vi "SortControlsColumn__slk_mt.vi"(8 "error in (no error)":errorcluster, 9 "Index":i32, 10 "Area Scale":T1, 11 "Controls":refnum<vi>[](array[refnum])) -> (0 "error out":errorcluster, 1 "Index":u32[](array[numeric]))   [LabVIEW 2015, in "Lazyboots Menu Tool.lvlib"]
uses:
  <vilib>/Utility/miscctls.llb/LVRectTypeDef.ctl
  <vilib>/SLK/Lazyboots Menu Tool/Library/Lazyboots Menu Tool.lvlib
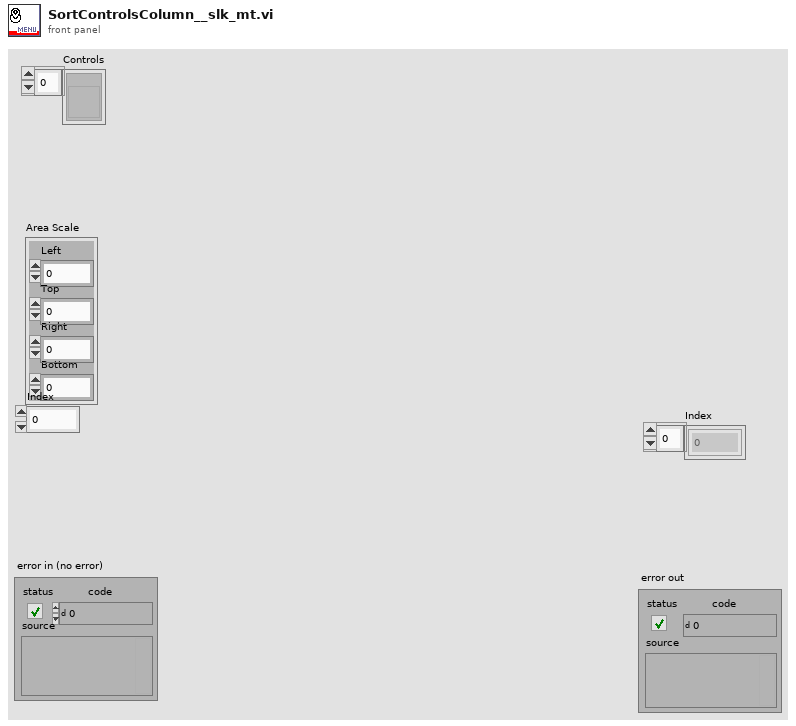
[diagram p1: front panel]
types:
  T1 = typedef "LVRectTypeDef.ctl" = cluster{"Left":i16, "Top":i16, "Right":i16, "Bottom":i16}
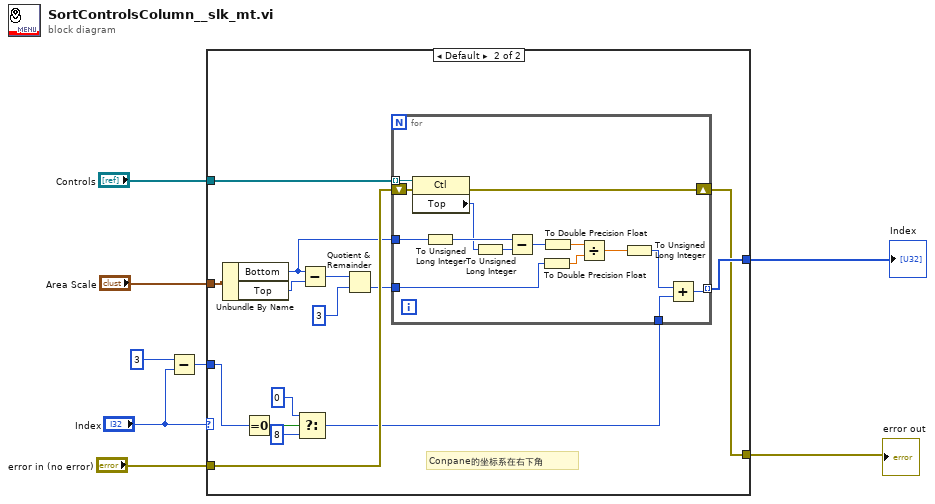
[diagram p0: block diagram]
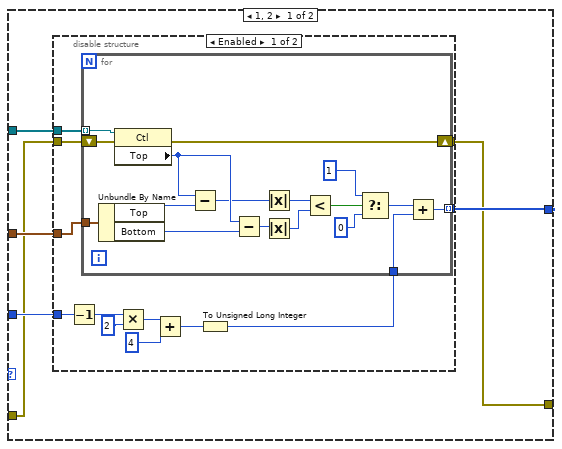
[diagram p2: hidden frame]
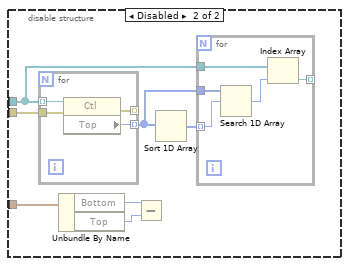
[diagram p3: hidden frame]
diagram:
  n1 = Subtract(x=3, y="Index") -> (x-y=w4:i32)
  n2 = case shown="Default" "Index" {
    tunnel: "Controls" -> [w13 w74]
    tunnel: "Area Scale" -> [w12 w73]
    tunnel: w4 -> [w14 w60]
    tunnel: [w11 w62] -> w1
    tunnel: "error in (no error)" -> [w10 w70]
    tunnel: [w9 w61] -> w2
    frame 1, 2 {
      n3 = disable-structure shown="Enabled" {
        disable-tunnel: w14 -> [w26 _]
        disable-tunnel: w13 -> [w21 w48]
        disable-tunnel: w12 -> [w20 w46]
        disable-tunnel: [w19 _] -> w11
        disable-tunnel: w10 -> [w18 w50]
        disable-tunnel: [w17 _] -> w9
        frame Enabled {
          n4 = Decrement(x=w26) -> (x-1=w25:i32)
          n5 = Multiply(x=w25, y=2) -> (x*y=w23:i32)
          n6 = Add(x=w23, y=4) -> (x+y=w16:i32)
          n7 = To Unsigned Long Integer(number=w16) -> (unsigned 32bit integer=w15:u32)
          n8 = for {
            tunnel: w21 -> [w43] mode=indexing
            tunnel: w20 -> [w42]
            tunnel: w15 -> [w30]
            tunnel: [w29] -> w19 mode=indexing
            shift-right: [w27] -> w17
            shift-left: w18 -> [w28]
            n9 = Unbundle By Name(w42) -> ("Top"=w41:i16, "Bottom"=w39:i16)
            n10 = property class="Ctl"(reference=w43, error in=w28) -> (error out=w27:errorcluster, "Top"=w40:i32)  [unwired: 1 out]
            n11 = Subtract(x=w40, y=w41) -> (x-y=w38:i32)
            n12 = Subtract(x=w40, y=w39) -> (x-y=w37:i32)
            n13 = Absolute Value(x=w38) -> (abs(x)=w36:i32)
            n14 = Absolute Value(x=w37) -> (abs(x)=w35:i32)
            n15 = Less?(x=w36, y=w35) -> (x < y?=w34:bool)
            n16 = Select(t=u32 1, s=w34, f=u32 0) -> (s? t:f=w31:u32)
            n17 = Add(x=w31, y=w30) -> (x+y=w29:u32)
          }
        }
        frame Disabled {
          n18 = for {
            tunnel: w48 -> [w59] mode=indexing
            tunnel: w50 -> [w58]
            tunnel: [w57] -> w47 mode=indexing
            tunnel: [w56] -> _ mode=indexing
            n19 = property class="Ctl"(reference=w59, error in=w58) -> (error out=w56:errorcluster, "Top"=w57:i32)  [unwired: 1 out]
          }
          n20 = Unbundle By Name(w46) -> ("Bottom"=w45:i16, "Top"=w44:i16)
          n21 = Subtract(x=w45, y=w44) -> ()  [unwired: 1 out]
          n22 = Sort 1D Array(array=w47) -> (sorted array=w49:i32[])
          n23 = for {
            tunnel: w49 -> [w54] mode=indexing
            tunnel: w48 -> [w53]
            tunnel: w47 -> [w55]
            tunnel: [w51] -> _ mode=indexing
            n24 = Search 1D Array(1D array=w55, element=w54) -> (index of element=w52:i32)  [unwired: 1 in]
            n25 = Index Array(array=w53, index=w52) -> (element=w51:refnum<vi>)
          }
        }
      }
    }
    frame Default {
      # "Conpane的坐标系在右下角"
      n26 = Unbundle By Name(w73) -> ("Bottom"=w67:i16, "Top"=w68:i16)
      n27 = Equal To 0?(x=w60) -> (x = 0?=w66:bool)
      n28 = Select(t=u32 0, s=w66, f=u32 8) -> (s? t:f=w63:u32)
      n29 = Subtract(x=w67, y=w68) -> (x-y=w72:i16)
      n30 = Quotient & Remainder(x=w72, y=i16 3) -> (floor(x/y)=w69:i16)  [unwired: 1 out]
      n31 = for {
        tunnel: w74 -> [w89] mode=indexing
        tunnel: w69 -> [w78]
        tunnel: w67 -> [w84]
        tunnel: w63 -> [w85]
        tunnel: [w87] -> w62 mode=indexing
        shift-right: [w86] -> w61
        shift-left: w70 -> [w88]
        n32 = property class="Ctl"(reference=w89, error in=w88) -> (error out=w86:errorcluster, "Top"=w81:i32)  [unwired: 1 out]
        n33 = To Unsigned Long Integer(number=w84) -> (unsigned 32bit integer=w83:u32)
        n34 = To Unsigned Long Integer(number=w81) -> (unsigned 32bit integer=w82:u32)
        n35 = Subtract(x=w83, y=w82) -> (x-y=w80:u32)
        n36 = To Double Precision Float(number=w78) -> (double precision float=w77:dbl)
        n37 = To Double Precision Float(number=w80) -> (double precision float=w79:dbl)
        n38 = Divide(x=w79, y=w77) -> (x/y=w76:dbl)
        n39 = To Unsigned Long Integer(number=w76) -> (unsigned 32bit integer=w75:u32)
        n40 = Add(x=w75, y=w85) -> (x+y=w87:u32)
      }
    }
  }
  "error out" <- w2
  "Index" <- w1
